vi "rosinterface.vi"() -> ()   [LabVIEW 2018]
uses:
  <vilib>/Tufts CEEO ROS for LabVIEW Software/ROS/Code/SubVIs/_ROSControl.ctl
  <vilib>/Tufts CEEO ROS for LabVIEW Software/ROS/Code/SubVIs/_ROSDirection.ctl
  <vilib>/Tufts CEEO ROS for LabVIEW Software/ROS/Code/Console/Servers/ServerSubs/TopicDef.ctl
  <vilib>/Tufts CEEO ROS for LabVIEW Software/ROS/MessageBuilding/std_msgs/subs/stringScalar.vi
  <vilib>/Tufts CEEO ROS for LabVIEW Software/ROS/MessageParsing/std_msgs/subs/parse_string_scalar.vi
panel:
  in  "table 6":bool
  out "ROS out 2":T1={"topic port"=0, "Node"="", "topic"="", "type"="", "node port"=0, "error "={"status"=FALSE, "code"=0, "source"=""}, "Direction"=enum."Node", "Update (ms)"=1, "FIFO size"=1}
  in  "table 5":bool
  in  "table 4":bool
  in  "table 3":bool
  in  "table2":bool
  in  "table 1":bool
  out "ROS out":T1={"topic port"=0, "Node"="", "topic"="", "type"="", "node port"=0, "error "={"status"=FALSE, "code"=0, "source"=""}, "Direction"=enum."Node", "Update (ms)"=1, "FIFO size"=1}
  in  "stop":bool
  out "Table  5":bool
  out "Table  4":bool
  out "Table  3":bool
  out "Table  2":bool
  out "Table 1":bool
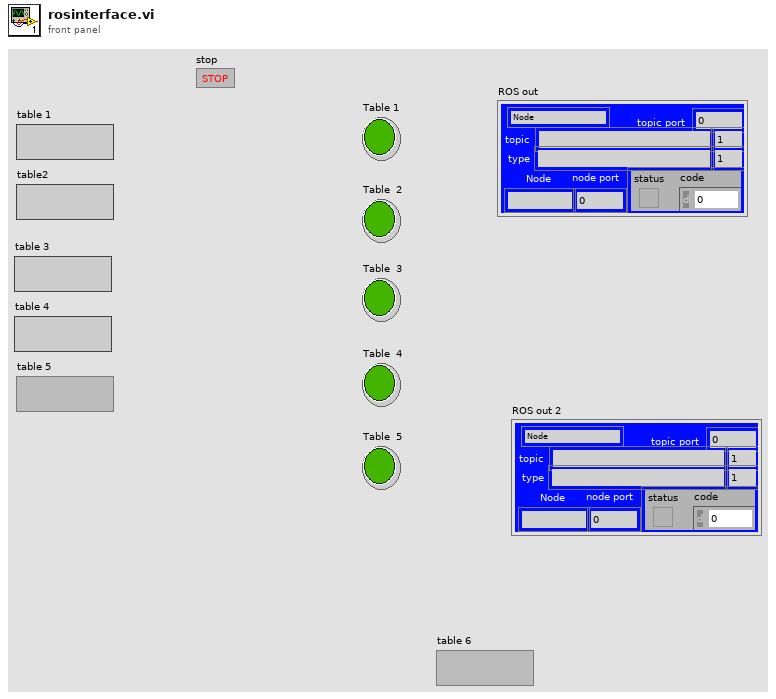
[diagram p1: front panel]
types:
  T1 = typedef "_ROSControl.ctl" = cluster{"topic port":u16, "Node":string, "topic":string, "type":string, "node port":u16, "error ":errorcluster, "Direction":T2, "Update (ms)":u16, "FIFO size":u16}
  T2 = typedef "_ROSDirection.ctl" = enum16{"Node", "Publisher", "Subscriber", "ServiceClient", "ServiceProvider"}
  T3 = typedef "TopicDef.ctl" = cluster{"Topic":string, "Type":string, "Action":T2, "Update (ms)":u16, "queue size":u16}
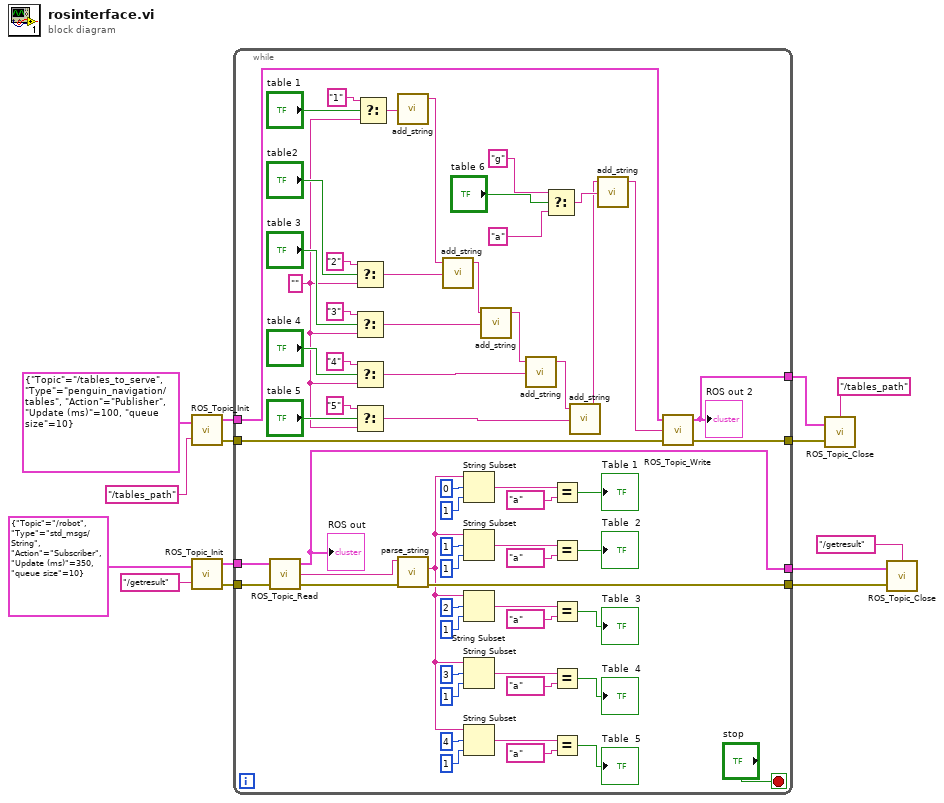
[diagram p0: block diagram]
diagram:
  n1 = call <vilib>:"ROS_Topic_Init.vi"("Definitions"=T3 {"Topic"="/tables_to_serve", "Type"="penguin_navigation/tables", "Action"=enum."Publisher", "Update (ms)"=100, "queue size"=10}, "node"="/tables_path") -> ("ROS out"=w6:T1, "error out"=w7:errorcluster)  [unwired: 1 in]
  n2 = call <vilib>:"ROS_Topic_Init.vi"("Definitions"=T3 {"Topic"="/robot", "Type"="std_msgs/String", "Action"=enum."Subscriber", "Update (ms)"=350, "queue size"=10}, "node"="/getresult") -> ("ROS out"=w13:T1, "error out"=w12:errorcluster)  [unwired: 1 in]
  n3 = while {
    tunnel: w13 -> [w77]
    tunnel: [w75] -> w9
    tunnel: w12 -> [w76]
    tunnel: [w74] -> w8
    tunnel: w6 -> [w58]
    tunnel: [w56] -> w4
    tunnel: w7 -> [w59]
    tunnel: [w57] -> w5
    stop <- "stop" stop-if-true
    w55 = "" ("t")
    n4 = call <vilib>:"ROS_Topic_Read.vi"("error in (no error)"=w76, "ROS in"=w77) -> ("error out"=w38:errorcluster, "Reply"=w39:string, "ROS out"=w75:T1)  [unwired: 1 in]
    "ROS out" <- w75
    n5 = Select(t="2", s="table2", f=w55) -> (s? t:f=w69:string)
    n6 = Select(t="3", s="table 3", f=w55) -> (s? t:f=w70:string)
    n7 = Select(t="4", s="table 4", f=w55) -> (s? t:f=w71:string)
    n8 = Select(t="5", s="table 5", f=w55) -> (s? t:f=w72:string)
    n9 = Select(t="1", s="table 1", f=w55) -> (s? t:f=w66:string)
    n10 = call-poly <vilib>:"add_string.vi"("String"=w66) -> ("msg out"=w67:string)  [unwired: 4 in]
    n11 = call-poly <vilib>:"parse_string.vi"("error in"=w38, "msg in"=w39) -> ("error out"=w74:errorcluster, "string"=w23:string)  [unwired: 3 in, 1 out]
    n12 = call-poly <vilib>:"add_string.vi"("String"=w69, "msg in"=w67) -> ("msg out"=w68:string)  [unwired: 3 in]
    n13 = String Subset(string=w23, offset (0)=0, length (rest)=1 ("offset (0)")) -> (substring=w37:string)
    n14 = String Subset(string=w23, offset (0)=1, length (rest)=1 ("offset (0)")) -> (substring=w36:string)
    n15 = String Subset(string=w23, offset (0)=2, length (rest)=1 ("offset (0)")) -> (substring=w35:string)
    n16 = String Subset(string=w23, offset (0)=3, length (rest)=1 ("offset (0)")) -> (substring=w34:string)
    n17 = String Subset(string=w23, offset (0)=4, length (rest)=1 ("offset (0)")) -> (substring=w33:string)
    n18 = call-poly <vilib>:"add_string.vi"("String"=w70, "msg in"=w68) -> ("msg out"=w65:string)  [unwired: 3 in]
    n19 = call-poly <vilib>:"add_string.vi"("String"=w71, "msg in"=w65) -> ("msg out"=w73:string)  [unwired: 3 in]
    n20 = Select(t="g", s="table 6", f="a") -> (s? t:f=w17:string)
    n21 = Equal?(x=w37, y="a") -> (x = y?=→"Table 1":bool)
    n22 = Equal?(x=w36, y="a") -> (x = y?=→"Table  2":bool)
    n23 = Equal?(x=w35, y="a") -> (x = y?=→"Table  3":bool)
    n24 = Equal?(x=w34, y="a") -> (x = y?=→"Table  4":bool)
    n25 = Equal?(x=w33, y="a") -> (x = y?=→"Table  5":bool)
    n26 = call-poly <vilib>:"add_string.vi"("String"=w72, "msg in"=w73) -> ("msg out"=w16:string)  [unwired: 3 in]
    n27 = call-poly <vilib>:"add_string.vi"("String"=w17, "msg in"=w16) -> ("msg out"=w15:string)  [unwired: 3 in]
    n28 = call <vilib>:"ROS_Topic_Write.vi"("error in (no error)"=w59, "Msg in"=w15, "ROS in"=w58) -> ("error out"=w57:errorcluster, "ROS out"=w56:T1)  [unwired: 1 in]
    "ROS out 2" <- w56
  }
  n29 = call <vilib>:"ROS_Topic_Close.vi"("error in"=w5, "ROS in"=w4, "node"="/tables_path") -> ()  [unwired: 1 in, 1 out]
  n30 = call <vilib>:"ROS_Topic_Close.vi"("error in"=w8, "ROS in"=w9, "node"="/getresult") -> ()  [unwired: 1 in, 1 out]
